vi "send request, get response.vi"(8 "error in (no error)":errorcluster, 10 "request":string, 11 "zmq_socket in":refnum<class "zmq_socket.lvclass">) -> (0 "error out":errorcluster, 1 "response":string, 2 "timeout?":bool, 3 "zmq_socket out":refnum<class "zmq_socket.lvclass">, 5 "more?":bool)   [LabVIEW 2018, in "LV-Julia_ZMQ-Roundtrip_lib.lvlib"]
uses:
  LV-Julia_ZMQ-Roundtrip_lib.lvlib
  <vilib>/addons/zeromq/zmq_socket.lvclass
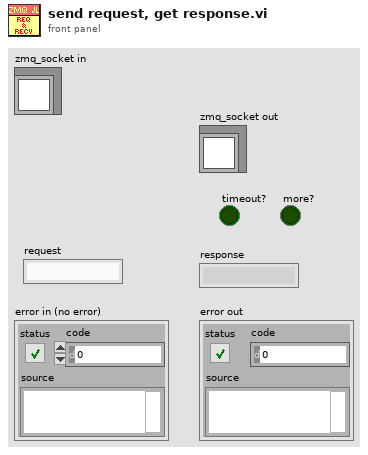
[diagram p1: front panel]
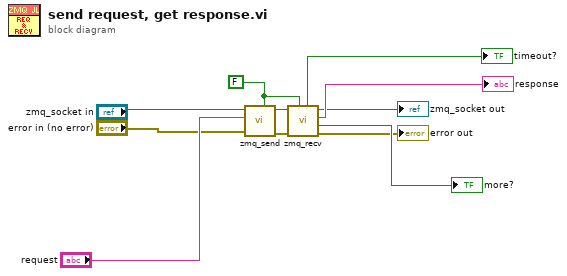
[diagram p0: block diagram]
diagram:
  w9 = FALSE ("more? (F)")
  n1 = call <vilib>:"zmq_send.vi"("error in"="error in (no error)", "data"="request", "socket in"="zmq_socket in", "more? (F)"=w9) -> ("error out"=w6:errorcluster, "socket out"=w3:refnum<class "zmq_socket.lvclass">)  [unwired: 3 in]
  n2 = call <vilib>:"zmq_recv.vi"("no block? (F)"=w9, "error in"=w6, "socket in"=w3) -> ("error out"=→"error out":errorcluster, "more?"=→"more?":bool, "data"=→"response":string, "socket out"=→"zmq_socket out":refnum<class "zmq_socket.lvclass">, "timeout?"=→"timeout?":bool)  [unwired: 2 in]
